vi "SerialChart.vi"() -> ()   [LabVIEW 2015]
uses:
  <vilib>/Instr/_visa.llb/VISA Configure Serial Port (Serial Instr).vi
panel:
  in  "清空缓冲区":bool
  in  "清空波形":bool
  out "C1":dbl
  out "C2":dbl
  out "C3":dbl
  out "缓冲区字节":u32
  in  "波特率":u16(ring)=1 items=["4800", "9600", "115200", "230400", "460800"]
  out "串口状态":bool
  in  "打开串口":bool
  in  "端口号":u16(ring) items=["COM1", "COM2", "COM3", "COM4", "COM5", "COM6"]
  in  "?":enum32{"独立波形图", "混合波形图"}(tab)
  out "幅值 C1":dbl(graph)
  out "幅值 C2":dbl(graph)
  out "幅值 C3":dbl(graph)
  out "幅值":dynamicdata(graph)
  out "关串口等待":u32=500
  in  "延时":u32
  out "VISA resource name":refnum<visa-resource-name> caption="VISA资源名称"
  # "SimpleOscillograph"
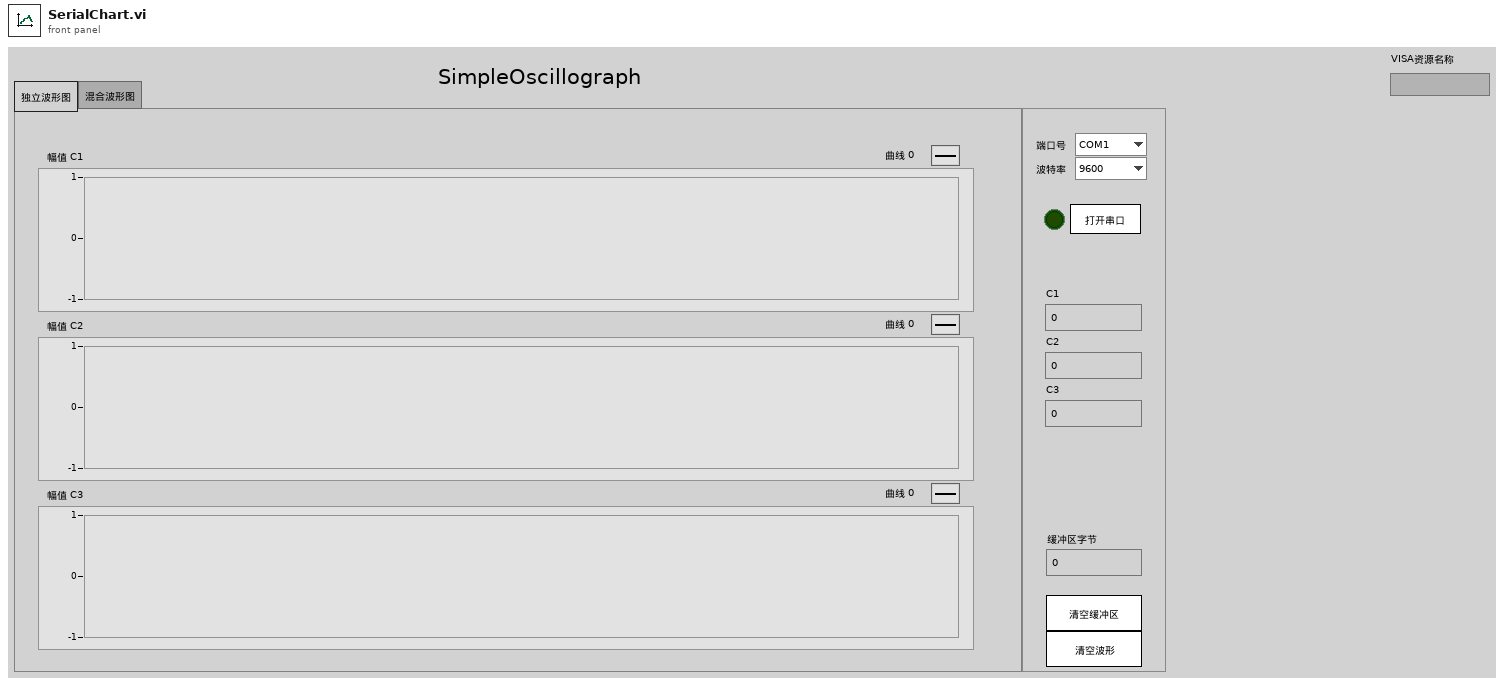
[diagram p1: front panel]
types:
  T1 = enum8{"Enabled", "Disabled", "Disabled and Grayed Out"}
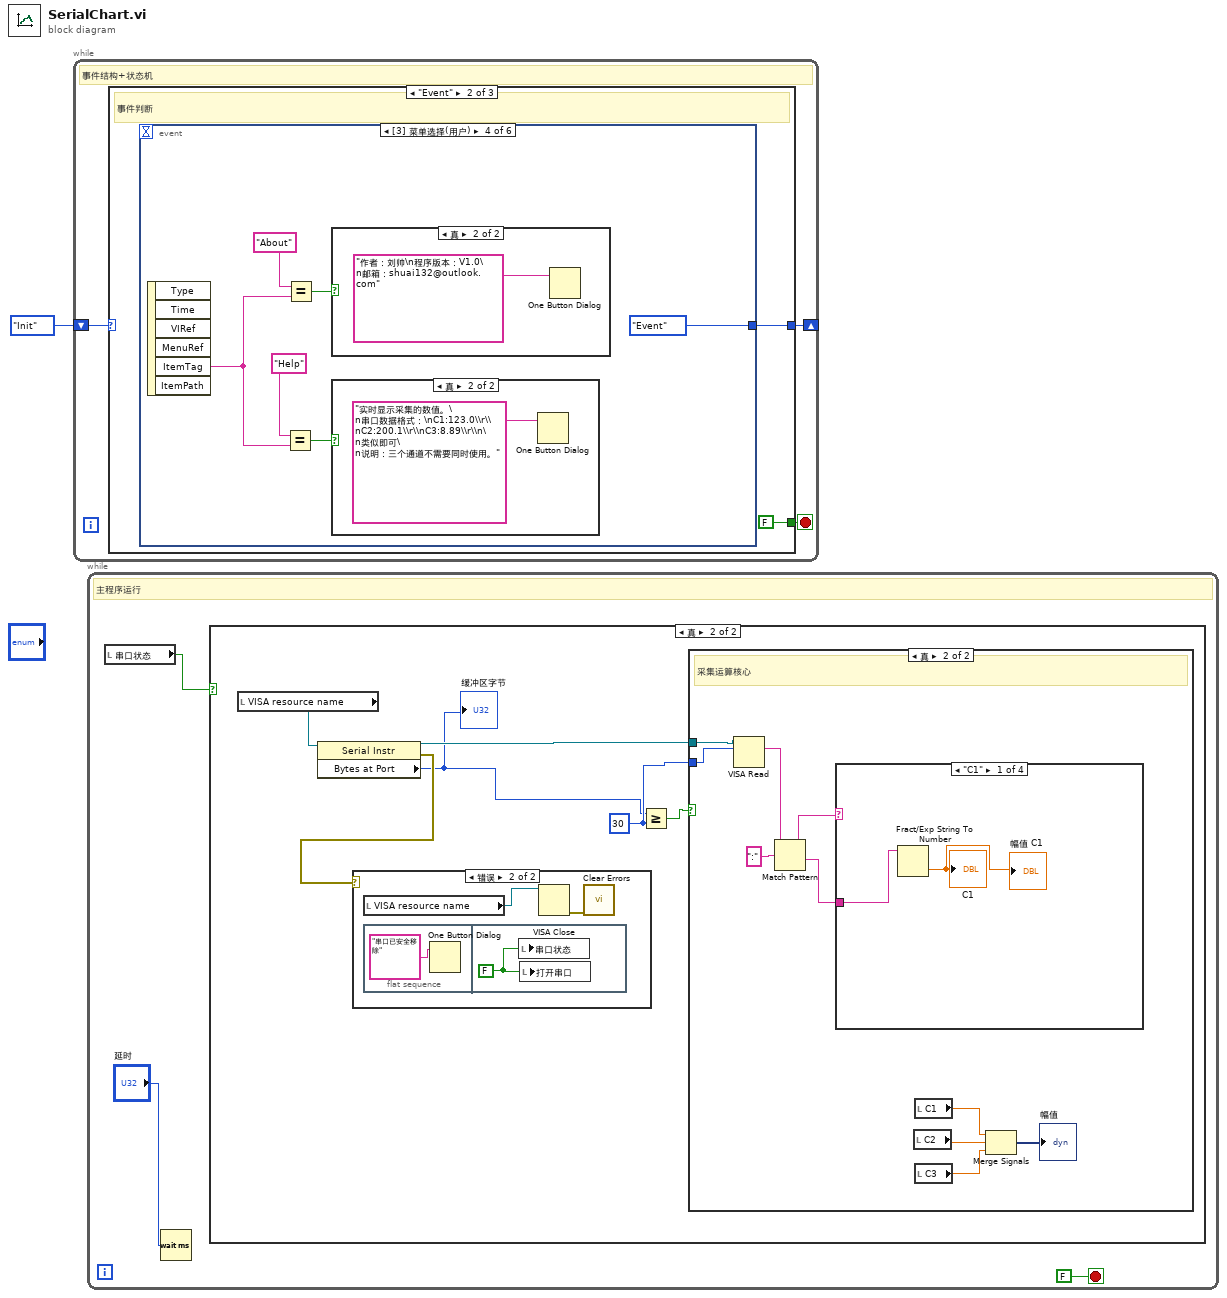
[diagram p0: block diagram]
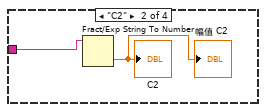
[diagram p5: hidden frame]
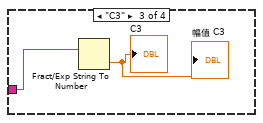
[diagram p6: hidden frame]
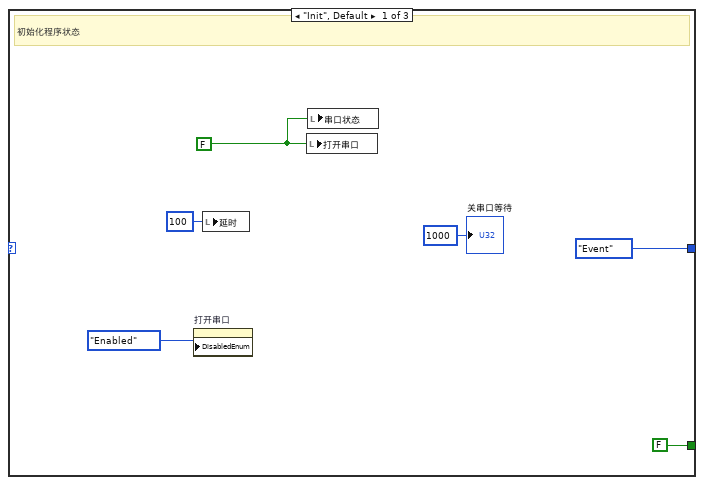
[diagram p8: hidden frame]
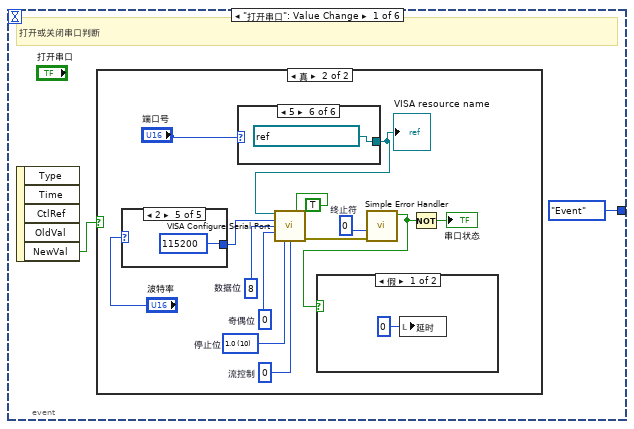
[diagram p9: hidden frame]
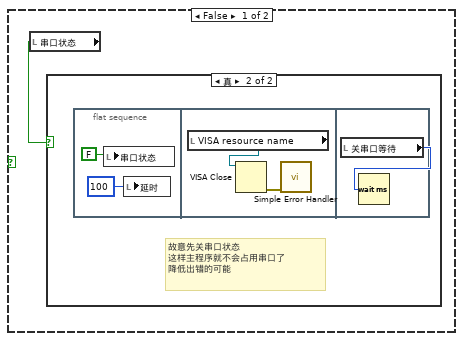
[diagram p10: hidden frame]
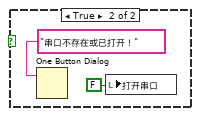
[diagram p12: hidden frame]
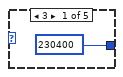
[diagram p13: hidden frame]
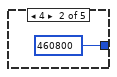
[diagram p14: hidden frame]
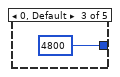
[diagram p15: hidden frame]
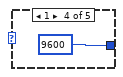
[diagram p16: hidden frame]
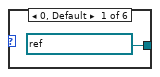
[diagram p17: hidden frame]
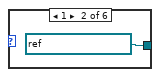
[diagram p18: hidden frame]
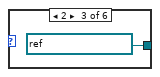
[diagram p19: hidden frame]
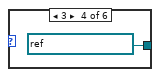
[diagram p20: hidden frame]
diagram:
  n1 = while {
    shift-right: [w2] -> _
    shift-left: enum16{"Init", "Event", "Exit"}."Init" -> [w3]
    stop <- w4 stop-if-true
    # "事件结构+状态机"
    n2 = case shown="\"Event\"" w3 {
      tunnel: [FALSE FALSE TRUE] -> w4
      tunnel: [enum16{"Init", "Event", "Exit"}."Event" w11 enum16{"Init", "Event", "Exit"}."Exit"] -> w2
      frame "Init", Default {
        w9 = FALSE ("exit")
        # "初始化程序状态"
        n3 = property on="打开串口" class="Bool (严格)"("DisabledEnum"=T1."Enabled" ("禁用")) -> ()  [unwired: 2 in, 2 out]
        n4 = local write "延时"(u32 100 ("延时")) -> ()
        n5 = local write "打开串口"(w9) -> ()
        n6 = local write "串口状态"(w9) -> ()
        "关串口等待" <- u32 1000 ("关串口等待")
      }
      frame "Event" {
        # "事件判断"
        n7 = event shown="[3] 菜单选择(用户)" {
          selector: _ -> [_ _ _ _ _ _]
          dyn-events: _ -> [_ _ _ _ _ _]
          timeout: _ -> [_ _ _ _ _ _]
          tunnel: [enum16{"Init", "Event", "Exit"}."Event" enum16{"Init", "Event", "Exit"}."Event" enum16{"Init", "Event", "Exit"}."Event" enum16{"Init", "Event", "Exit"}."Event" enum16{"Init", "Event", "Exit"}."Event" enum16{"Init", "Event", "Exit"}."Exit"] -> w11
          event "打开串口": Value Change {
            # "打开或关闭串口判断"
            n8 = event-data() -> ("NewVal"=w13:bool)  [unwired: 1 in, 4 out]
            n9 = case shown="真" w13 {
              frame False {
                n10 = local read "串口状态"() -> (w15:bool)
                n11 = case shown="真" w15 {
                  frame False {
                  }
                  frame True {
                    # "故意先关串口状态\n这样主程序就不会占用串口了\n降低出错的可能"
                    n12 = flat-sequence {
                      frame #0 {
                        n13 = local write "串口状态"(FALSE) -> ()
                        n14 = local write "延时"(u32 100 ("延时")) -> ()
                      }
                      frame #1 {
                        n15 = local read "VISA resource name"() -> (w18:refnum<visa-resource-name>)
                        n16 = VISA Close(VISA resource name=w18) -> (error out=w19:errorcluster)  [unwired: 1 in]
                        n17 = call <vilib>:"Simple Error Handler.vi"("error in (no error)"=w19) -> ()  [unwired: 4 in, 5 out]
                      }
                      frame #2 {
                        n18 = local read "关串口等待"() -> (w20:u32)
                        n19 = Wait (ms)(milliseconds to wait=w20) -> ()  [unwired: 1 out]
                      }
                    }
                  }
                }
              }
              frame True {
                w21 = u16 10 items=["1.0"=10, "1.5"=15, "2.0"=20]  # 停止位
                w25 = TRUE  # 终止符
                w31 = u16 0  # 流控制
                w30 = u8 0  # 奇偶位
                w29 = u16 8  # 数据位
                n20 = case shown="2" "波特率" {
                  tunnel: [230400 460800 4800 9600 115200] -> w28
                  frame 3 {
                  }
                  frame 4 {
                  }
                  frame 0, Default {
                  }
                  frame 1 {
                  }
                  frame 2 {
                  }
                }
                n21 = case shown="5" "端口号" {
                  tunnel: [refnum<visa-resource-name> "ASRL1::INSTR" ("VISA resource name") refnum<visa-resource-name> "ASRL2::INSTR" ("VISA resource name") refnum<visa-resource-name> "ASRL3::INSTR" ("VISA resource name") refnum<visa-resource-name> "ASRL4::INSTR" ("VISA resource name") refnum<visa-resource-name> "ASRL5::INSTR" ("VISA resource name") refnum<visa-resource-name> "ASRL6::INSTR" ("VISA resource name")] -> w22
                  frame 0, Default {
                  }
                  frame 1 {
                  }
                  frame 2 {
                  }
                  frame 3 {
                  }
                  frame 4 {
                  }
                  frame 5 {
                  }
                }
                "VISA resource name" <- w22
                n22 = call-poly "VISA Configure Serial Port"("VISA resource name"=w22, "Enable Termination\nChar (T)"=w25, "baud rate (9600)"=w28, "data bits (8)"=w29, "parity (0:none)"=w30, "stop bits (10: 1 bit)"=w21, "flow control (0:none)"=w31) -> ("error out"=w32:errorcluster)  [unwired: 7 in, 1 out]
                n23 = call <vilib>:"Simple Error Handler.vi"("type of dialog (OK msg:1)"=0, "error in (no error)"=w32) -> ("error?"=w26:bool)  [unwired: 3 in, 4 out]
                n24 = case shown="假" w26 {
                  frame False {
                    n25 = local write "延时"(u32 0 ("延时")) -> ()
                  }
                  frame True {
                    n26 = One Button Dialog(message="串口不存在或已打开！") -> ()  [unwired: 1 in, 1 out]
                    n27 = local write "打开串口"(FALSE) -> ()
                  }
                }
                n28 = Not(x=w26) -> (.not. x?=→"串口状态":bool)
              }
            }
          }
          event "端口号", "波特率": Value Change {
            n29 = event-data() -> ("OldVal"=w49:u16)  [unwired: 1 in, 4 out]
            n30 = local read "串口状态"() -> (w50:bool)
            n31 = case shown="真" w50 {
              tunnel: w49 -> [_ w51]
              frame False {
              }
              frame True {
                n32 = flat-sequence {
                  tunnel: w51 -> [w56]
                  frame #0 {
                    n33 = case shown="0, 默认" w56 {
                      tunnel: [refnum<visa-resource-name> "ASRL1::INSTR" ("VISA resource name") refnum<visa-resource-name> "ASRL2::INSTR" ("VISA resource name") refnum<visa-resource-name> "ASRL3::INSTR" ("VISA resource name") refnum<visa-resource-name> "ASRL4::INSTR" ("VISA resource name") refnum<visa-resource-name> "ASRL5::INSTR" ("VISA resource name")] -> w53
                      frame 0, Default {
                      }
                      frame 1 {
                      }
                      frame 2 {
                      }
                      frame 3 {
                      }
                      frame 4 {
                      }
                    }
                    n34 = VISA Close(VISA resource name=w53) -> (error out=w55:errorcluster)  [unwired: 1 in]
                    n35 = call <vilib>:"Simple Error Handler.vi"("error in (no error)"=w55) -> ()  [unwired: 4 in, 5 out]
                    n36 = local write "串口状态"(FALSE) -> ()
                    n37 = local write "打开串口"(FALSE ("open")) -> ()
                  }
                }
              }
            }
          }
          event "清空缓冲区": Value Change {
            n38 = event-data() -> ()  [unwired: 1 in, 6 out]
            n39 = local read "串口状态"() -> (w62:bool)
            n40 = case shown="假" w62 {
              frame False {
                n41 = call "显示对话框信息"() -> ()  [unwired: 10 in, 2 out]
              }
              frame True {
                n42 = local read "VISA resource name"() -> (w64:refnum<visa-resource-name>)
                n43 = VISA Flush I/O Buffer(VISA resource name=w64) -> ()  [unwired: 2 in, 2 out]
              }
            }
          }
          event Menu Selection (User) {
            n44 = event-data() -> ("ItemTag"=w68:string)  [unwired: 1 in, 5 out]
            n45 = Equal?(x="Help", y=w68) -> (x = y?=w69:bool)
            n46 = Equal?(x="About", y=w68) -> (x = y?=w70:bool)
            n47 = case shown="真" w70 {
              frame False {
              }
              frame True {
                n48 = One Button Dialog(message="作者：刘帅\n程序版本：V1.0\n邮箱：shuai132@outlook.com" ("Message")) -> ()  [unwired: 1 in, 1 out]
              }
            }
            n49 = case shown="真" w69 {
              frame False {
              }
              frame True {
                n50 = One Button Dialog(message="实时显示采集的数值。\n串口数据格式：\nC1:123.0\\r\\nC2:200.1\\r\\nC3:8.89\\r\\n\n类似即可\n说明：三个通道不需要同时使用。" ("Message")) -> ()  [unwired: 1 in, 1 out]
              }
            }
          }
          event "清空波形": Value Change {
            w74 = dbl[] [] ("历史数据")
            n51 = event-data() -> ()  [unwired: 1 in, 6 out]
            n52 = property on="幅值" class="WFChart (严格)"("History Data"=dynamicdata[] [] ("历史数据")) -> ()  [unwired: 2 in, 2 out]
            n53 = property on="幅值 C3" class="WFChart (严格)"("History Data"=w74) -> ()  [unwired: 2 in, 2 out]
            n54 = property on="幅值 C2" class="WFChart (严格)"("History Data"=w74) -> ()  [unwired: 2 in, 2 out]
            n55 = property on="幅值 C1" class="WFChart (严格)"("History Data"=w74) -> ()  [unwired: 2 in, 2 out]
          }
          event Application Instance Close {
            # "退出程序"
            n56 = event-data() -> ()  [unwired: 1 in, 4 out]
            n57 = local read "串口状态"() -> (w77:bool)
            n58 = case shown="真" w77 {
              frame False {
              }
              frame True {
                # "故意先关串口状态\n这样主程序就不会占用串口了\n降低出错的可能"
                n59 = flat-sequence {
                  frame #0 {
                    n60 = local write "串口状态"(FALSE) -> ()
                    n61 = local write "延时"(u32 100 ("延时")) -> ()
                  }
                  frame #1 {
                    n62 = local read "VISA resource name"() -> (w80:refnum<visa-resource-name>)
                    n63 = VISA Close(VISA resource name=w80) -> (error out=w81:errorcluster)  [unwired: 1 in]
                    n64 = call <vilib>:"Simple Error Handler.vi"("error in (no error)"=w81) -> ()  [unwired: 4 in, 5 out]
                  }
                  frame #2 {
                    n65 = local read "关串口等待"() -> (w82:u32)
                    n66 = Wait (ms)(milliseconds to wait=w82) -> ()  [unwired: 1 out]
                  }
                }
              }
            }
          }
        }
      }
      frame "Exit" {
        # "退出前要处理的内容"
      }
    }
  }
  n67 = while {
    stop <- FALSE stop-if-true
    # "主程序运行"
    n68 = local read "串口状态"() -> (w87:bool)
    n69 = Wait (ms)(milliseconds to wait="延时") -> ()  [unwired: 1 out]
    n70 = case shown="真" w87 {
      frame False {
      }
      frame True {
        w89 = u32 30 ("y")
        n71 = local read "VISA resource name"() -> (w93:refnum<visa-resource-name>)
        n72 = property class="Serial Instr"(reference=w93) -> (reference out=w92:refnum<visa-resource-name>, error out=w91:errorcluster, "Bytes at Port"=w88:u32)  [unwired: 1 in]
        "缓冲区字节" <- w88
        n73 = case shown="错误" w91 {
          frame No Error {
          }
          frame Error {
            n74 = local read "VISA resource name"() -> (w94:refnum<visa-resource-name>)
            n75 = flat-sequence {
              frame #0 {
                n76 = One Button Dialog(message="串口已安全移除") -> ()  [unwired: 1 in, 1 out]
              }
              frame #1 {
                w97 = FALSE ("exit")
                n77 = local write "串口状态"(w97) -> ()
                n78 = local write "打开串口"(w97) -> ()
              }
            }
            n79 = VISA Close(VISA resource name=w94) -> (error out=w95:errorcluster)  [unwired: 1 in]
            n80 = call <vilib>:"Clear Errors.vi"("error in (no error)"=w95) -> ()  [unwired: 5 in, 2 out]
          }
        }
        n81 = Greater Or Equal?(x=w88, y=w89) -> (x >= y?=w90:bool)
        n82 = case shown="真" w90 {
          tunnel: w92 -> [_ w107]
          tunnel: w89 -> [_ w106]
          frame False {
          }
          frame True {
            # "采集运算核心"
            n83 = VISA Read(VISA resource name=w107, byte count=w106) -> (read buffer=w103:string)  [unwired: 1 in, 3 out]
            n84 = Match Pattern(string=w103, regular expression=":" ("正则表达式")) -> (before substring=w102:string, after substring=w104:string)  [unwired: 1 in, 2 out]
            n85 = case shown="\"C1\"" w102 {
              tunnel: w104 -> [w109 w111 w113 _]
              frame "C1" {
                n86 = Fract/Exp String To Number(string=w109) -> (number=→"C1" →"幅值 C1":dbl)  [unwired: 3 in, 1 out]
              }
              frame "C2" {
                n87 = Fract/Exp String To Number(string=w111) -> (number=→"C2" →"幅值 C2":dbl)  [unwired: 3 in, 1 out]
              }
              frame "C3" {
                n88 = Fract/Exp String To Number(string=w113) -> (number=→"C3" →"幅值 C3":dbl)  [unwired: 3 in, 1 out]
              }
              frame Default {
              }
            }
            n89 = local read "C2"() -> (w99:dbl)
            n90 = local read "C1"() -> (w100:dbl)
            n91 = local read "C3"() -> (w98:dbl)
            n92 = Merge Signals(w100, w99, w98) -> (→"幅值":dynamicdata)
          }
        }
      }
    }
  }
